vi "destroy.vi"(8 "error in (no error)":errorcluster, 11 "midi-file-events":refnum<class "midi-file-events.lvclass">) -> (0 "error out":errorcluster)   [LabVIEW 2020, in "midi-file-events.lvclass"]
uses:
  midi-file-events.lvclass
  midi-file-events.lvclass/midi-file-events.ctl
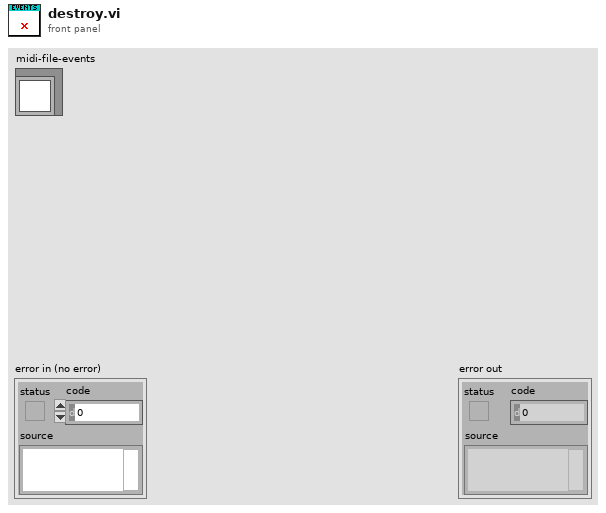
[diagram p1: front panel]
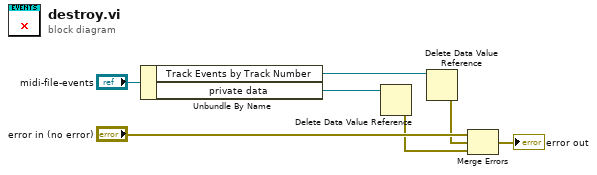
[diagram p0: block diagram]
diagram:
  n1 = Unbundle By Name("midi-file-events") -> ("Track Events by Track Number"=w6:refnum<data-value>, "private data"=w2:refnum<data-value>)
  n2 = Delete Data Value Reference(data value reference=w2) -> (error out=w1:errorcluster)  [unwired: 1 in, 1 out]
  n3 = Delete Data Value Reference(data value reference=w6) -> (error out=w4:errorcluster)  [unwired: 1 in, 1 out]
  n4 = Merge Errors("error in (no error)", w4, w1) -> (→"error out":errorcluster)
